vi "ArrangeValuesByName.vi"(10 "Names":string[](array[string]), 11 "Names/Values in":string[][](array[string])) -> (3 "Values Out":string[](array[string]))   [LabVIEW 2018]
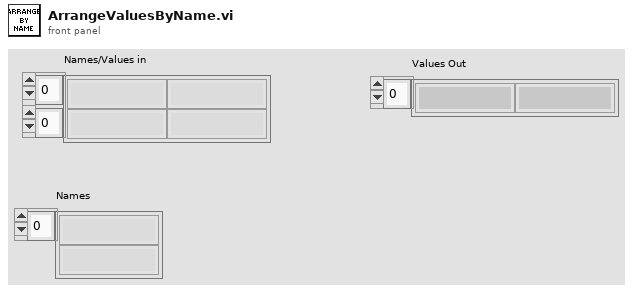
[diagram p1: front panel]
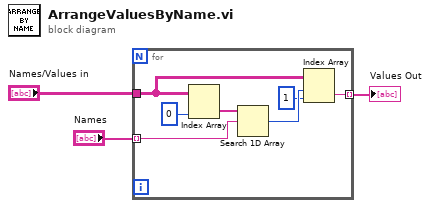
[diagram p0: block diagram]
diagram:
  n1 = for {
    tunnel: "Names" -> [w8] mode=indexing
    tunnel: "Names/Values in" -> [w6]
    tunnel: [w5] -> w1 mode=indexing
    n2 = Index Array(array=w6, index (col)=0 ("disabled index (col)")) -> (element=w9:string[])  [unwired: 1 in]
    n3 = Search 1D Array(1D array=w9, element=w8) -> (index of element=w7:i32)  [unwired: 1 in]
    n4 = Index Array(array=w6, index (row)=w7, index (col)=1 ("disabled index (col)")) -> (element=w5:string)
  }
  "Values Out" <- w1
